vi "Get Dependent Nodes from SysDef Root.vi"(8 "error in (no error)":errorcluster, 9 "GUID":string, 10 "Path":string, 11 "SysDef Ref":refnum<k24>) -> (0 "error out":errorcluster, 2 "Channels":string[](array[string]), 3 "Found":bool)   [LabVIEW 2019, in "Control Workspace Shared.lvlib"]
uses:
  NationalInstruments.VeriStand.SystemStorage
  Addon/Addon Shared/SubVIs/Constants.vi
  Control Workspace Shared.lvlib
  Addon/Addon Shared/Control Addon Shared.lvlib
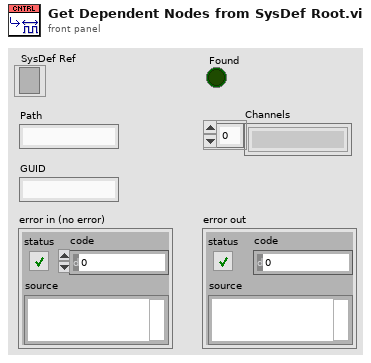
[diagram p1: front panel]
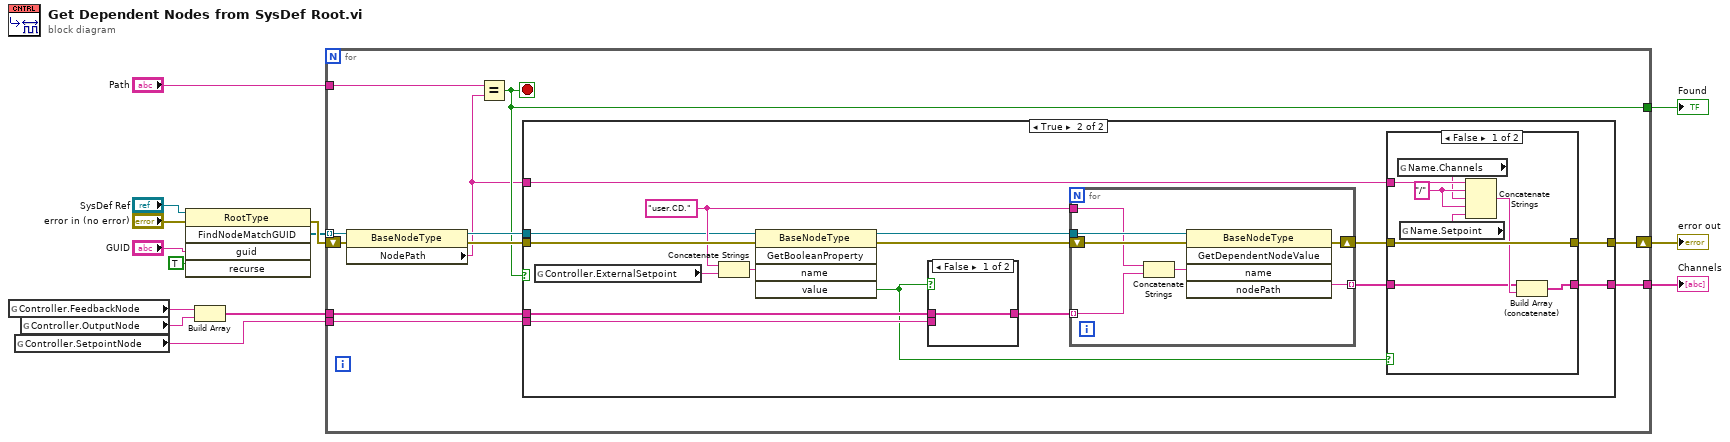
[diagram p0: block diagram]
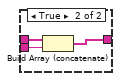
[diagram p4: hidden frame]
diagram:
  n1 = global read "Constants.vi" "Controller.FeedbackNode"() -> (w6:string)
  n2 = global read "Constants.vi" "Controller.SetpointNode"() -> (w1:string)
  n3 = global read "Constants.vi" "Controller.OutputNode"() -> (w7:string)
  n4 = invoke class="RootType" method="FindNodeMatchGUID"(reference="SysDef Ref", error in="error in (no error)", "guid"="GUID", "recurse"=TRUE) -> (error out=w9:errorcluster, "FindNodeMatchGUID"=w5:refnum<k24>[])  [unwired: 1 in, 3 out]
  n5 = Build Array(w6, w7) -> (w8:string[])
  n6 = for {
    tunnel: w5 -> [w24] mode=indexing
    tunnel: w8 -> [w25]
    shift-right: [w20] -> w13
    shift-left: w9 -> [w22]
    tunnel: [w18] -> w14
    tunnel: [w19] -> w12
    tunnel: "Path" -> [w16]
    tunnel: w1 -> [w17]
    stop <- w18 stop-if-true
    n7 = property class="BaseNodeType"(reference=w24, error in=w22) -> (reference out=w23:refnum<k24>, error out=w21:errorcluster, "NodePath"=w15:string)
    n8 = Equal?(x=w16, y=w15) -> (x = y?=w18:bool)
    n9 = case shown="True" w18 {
      tunnel: w25 -> [_ w37]
      tunnel: w23 -> [_ w27]
      tunnel: w21 -> [w26 w41]
      tunnel: [w26 w31] -> w20
      tunnel: [_ w29] -> w19
      tunnel: w17 -> [_ w36]
      tunnel: w15 -> [_ w28]
      frame False {
      }
      frame True {
        w34 = "user.CD." ("string")
        n10 = global read "Constants.vi" "Controller.ExternalSetpoint"() -> (w39:string)
        n11 = Concatenate Strings(w34, w39) -> (w38:string)
        n12 = invoke class="BaseNodeType" method="GetBooleanProperty"(reference=w27, error in=w41, "name"=w38) -> (reference out=w42:refnum<k24>, error out=w40:errorcluster, "value"=w33:bool)  [unwired: 2 in, 2 out]
        n13 = case shown="False" w33 {
          tunnel: w37 -> [w53 w56]
          tunnel: w36 -> [_ w55]
          tunnel: [w53 w54] -> w35
          frame False {
          }
          frame True {
            n14 = Build Array (concatenate)(w56, w55) -> (w54:string[])
          }
        }
        n15 = for {
          tunnel: w42 -> [w63]
          tunnel: w35 -> [w62] mode=indexing
          shift-right: [w60] -> w30
          shift-left: w40 -> [w61]
          tunnel: [w59] -> w32 mode=indexing
          tunnel: w34 -> [w58]
          n16 = Concatenate Strings(w58, w62) -> (w57:string)
          n17 = invoke class="BaseNodeType" method="GetDependentNodeValue"(reference=w63, error in=w61, "name"=w57) -> (error out=w60:errorcluster, "nodePath"=w59:string)  [unwired: 2 in, 3 out]
        }
        n18 = case shown="False" w33 {
          tunnel: w32 -> [w46 w51]
          tunnel: [w48 w52] -> w31
          tunnel: w30 -> [w48 w52]
          tunnel: [w45 w51] -> w29
          tunnel: w28 -> [w50 _]
          frame False {
            w44 = "/"
            n19 = global read "Constants.vi" "Name.Channels"() -> (w43:string)
            n20 = global read "Constants.vi" "Name.Setpoint"() -> (w49:string)
            n21 = Concatenate Strings(w50, w44, w43, w44, w49) -> (w47:string)
            n22 = Build Array (concatenate)(w46, w47) -> (w45:string[])
          }
          frame True {
          }
        }
      }
    }
  }
  "Found" <- w14
  "error out" <- w13
  "Channels" <- w12
